vi "בדיקת זמן ניתוק הממסר 4.vi"(7 "resultUserPrompt":bool, 8 "error":errorcluster, 11 "Path for Log":path) -> (0 "error out":errorcluster, 1 "בטוח כן/לא":bool, 2 "בדיקת זמן ניתוק הממסר":dbl)   [LabVIEW 2015]
uses:
  <instrlib>/niDMM/nidmm.llb/niDMM Function.ctl
  <instrlib>/niDMM/nidmm.llb/niDMM Resolution in Digits.ctl
  <vilib>/DAQmx/write.llb/DAQmx Write (Digital Bool 1Line 1Point).vi
  <vilib>/DAQmx/create/channels.llb/DAQmx Create Channel (DO-Digital Output).vi
  <vilib>/DAQmx/miscellaneous.llb/DAQmx Fill In Error Info.vi
  <instrlib>/niDMM/nidmm.llb/niDMM Configure Measurement Digits.vi
panel:
  in  "התחל":bool
  # "Right-Click to\nexplain error"
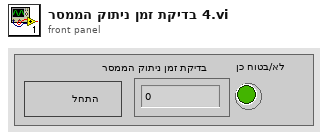
[diagram p1: front panel]
types:
  T1 = enum32{"Invalid", "Standard", "Closed", "Hidden", "Minimized", "Maximized"}
  T2 = typedef "niDMM Function.ctl" = enum16{"DC Volts", "AC Volts", "DC Current", "AC Current", "2-wire Resistance", "4-wire Resistance", "Diode", "Frequency", "Period", "AC Volts DC Coupled", "Capacitance", "Inductance", "Temperature"}
  T3 = typedef "niDMM Resolution in Digits.ctl" = dbl
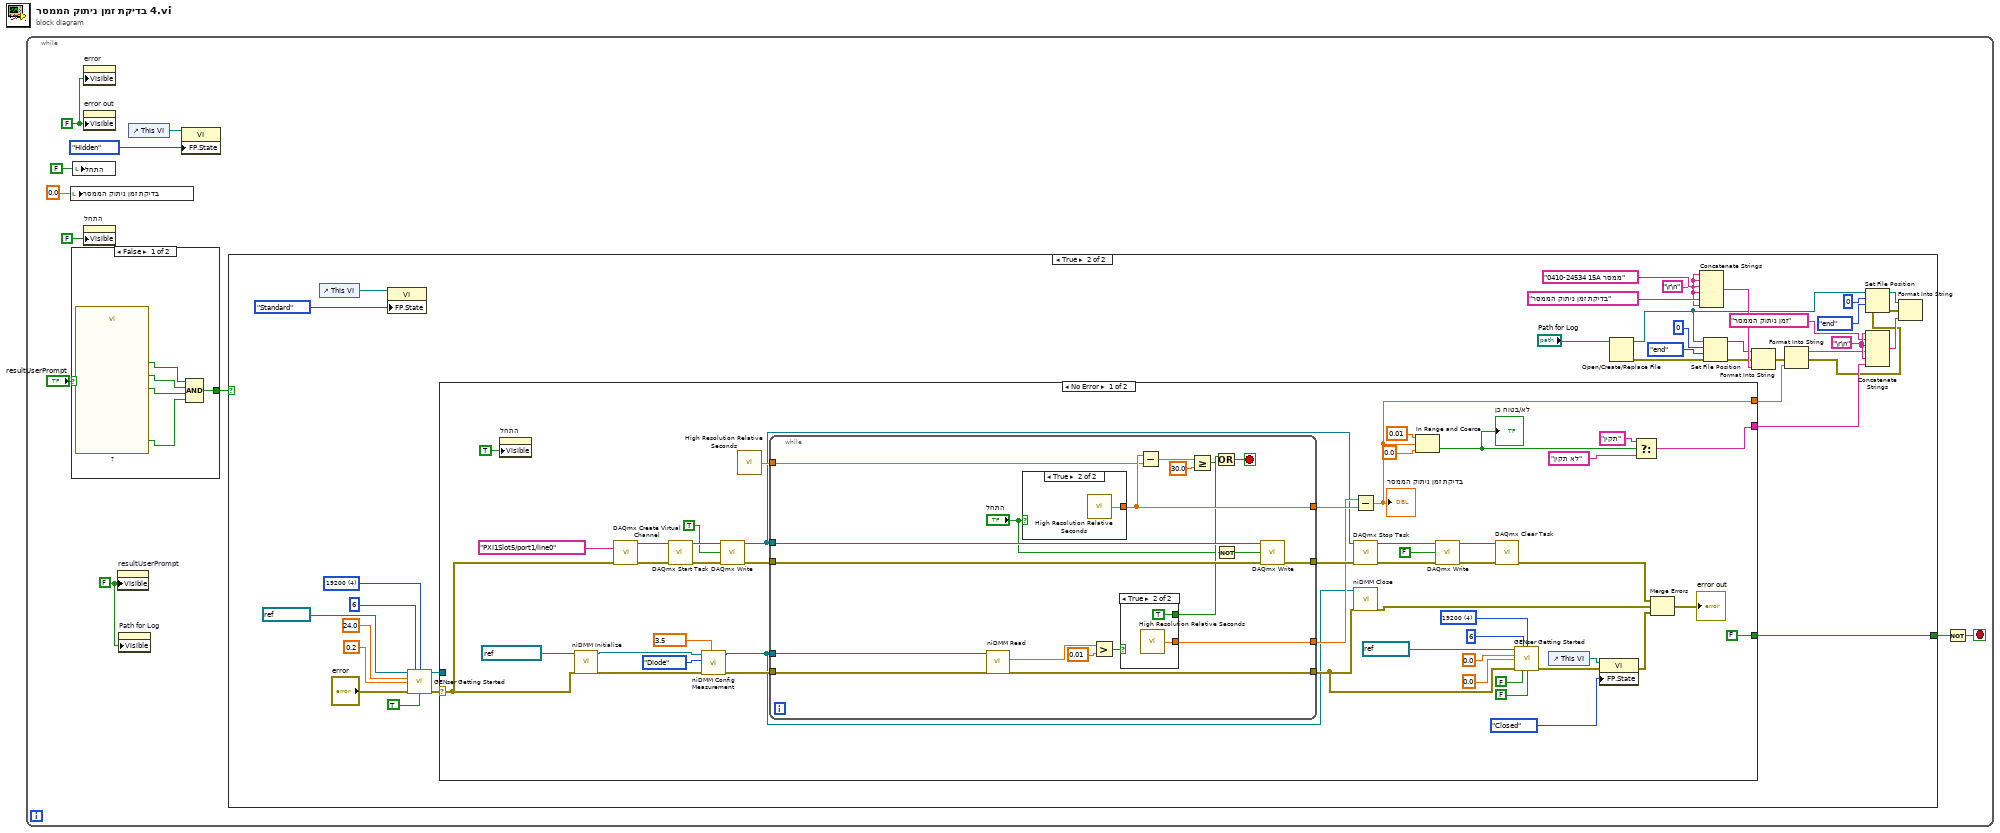
[diagram p0: block diagram]
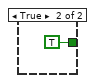
[diagram p2: hidden frame]
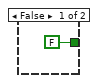
[diagram p3: hidden frame]
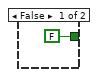
[diagram p4: hidden frame]
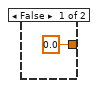
[diagram p5: hidden frame]
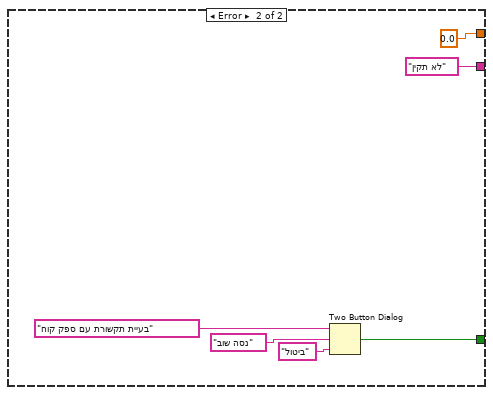
[diagram p6: hidden frame]
diagram:
  n1 = while {
    stop <- w10 stop-if-true
    w1 = FALSE ("Visible")
    w8 = FALSE ("Visible")
    n2 = local write "בדיקת זמן ניתוק הממסר"(0.0 ("זמן ניתוק הממסר")) -> ()
    n3 = case shown="False" "resultUserPrompt" {
      tunnel: [w16 TRUE] -> w11
      frame False {
        n4 = call "?"() -> ("הדקי הרב מודד"=w12:bool, "(מגע שלילי (מעטפת"=w13:bool, "A מגע חיובי"=w14:bool, "OK"=w15:bool)  [unwired: 15 in, 1 out]
        n5 = Compound Arithmetic op=AND(w15, w14, w13, w12) -> (w16:bool)
      }
      frame True {
      }
    }
    n6 = local write "התחל"(FALSE ("זמן ניתוק הממסר בטווח כן /לא")) -> ()
    n7 = property on="error" class="Clust (strict)"("Visible"=w8) -> ()  [unwired: 2 in, 2 out]
    n8 = property on="error out" class="Clust (strict)"("Visible"=w8) -> ()  [unwired: 2 in, 2 out]
    n9 = property on="התחל" class="Bool (strict)"("Visible"=FALSE) -> ()  [unwired: 2 in, 2 out]
    n10 = property on="resultUserPrompt" class="Bool (strict)"("Visible"=w1) -> ()  [unwired: 2 in, 2 out]
    n11 = property on="Path for Log" class="Path"("Visible"=w1) -> ()  [unwired: 2 in, 2 out]
    n12 = control-ref of="This VI"() -> (w7:refnum<vi>)
    n13 = property class="VI"(reference=w7, "FP.State"=T1."Hidden" ("Front Panel Window:State")) -> ()  [unwired: 1 in, 2 out]
    n14 = case shown="True" w11 {
      tunnel: [FALSE ("T button?") w46] -> w9
      frame False {
      }
      frame True {
        w27 = "\r\n"
        w35 = "\r\n"
        w50 = u16 4 items=["1200", "2400", "4800", "9600", "19200"] ("BAUD")
        n15 = control-ref of="This VI"() -> (w45:refnum<vi>)
        n16 = property class="VI"(reference=w45, "FP.State"=T1."Standard" ("Front Panel Window:State")) -> ()  [unwired: 1 in, 2 out]
        n17 = call "GENser Getting Started.vi"("VISA"=refnum<visa-resource-name> "COM6", "GEN Addr"=i16 6, "BAUD"=w50, "Voltage Limit"=24.0, "Current Limit"=0.2, "error"="error", "Output On (T)"=TRUE) -> ("VISA out"=w51:refnum<visa-resource-name>, "error out"=w42:errorcluster)  [unwired: 5 in, 2 out]
        n18 = case shown="No Error" w42 {
          selector: w42 -> [w56 _]
          tunnel: w51 -> [_ _]
          tunnel: [FALSE ("T button?") w129] -> w46
          tunnel: [w77 0.0] -> w21
          tunnel: [w73 "לא תקין"] -> w20
          frame No Error {
            w61 = T3 3.5 items=["3 1/2"=3.5, "4 1/2"=4.5, "5 1/2"=5.5, "6 1/2"=6.5, "7 1/2"=7.5] ("Resolution in Digits")
            w91 = u16 4 items=["1200", "2400", "4800", "9600", "19200"] ("BAUD")
            n19 = property on="התחל" class="Bool (strict)"("Visible"=TRUE) -> ()  [unwired: 2 in, 2 out]
            n20 = call <instrlib>:"niDMM Initialize.vi"("error in (no error)"=w56, "Instrument Descriptor"=refnum<k15> "PXI1Slot9") -> ("error out"=w58:errorcluster, "instrument handle out"=w59:refnum<k15>)  [unwired: 8 in]
            n21 = call-poly <vilib>:"DAQmx Create Virtual Channel.vi"("lines"=tag "PXI1Slot5/port1/line0", "error in"=w56) -> ("task out"=w70:refnum<k21>, "error out"=w71:errorcluster)  [unwired: 12 in]
            n22 = call <vilib>:"DAQmx Start Task.vi"("task/channels in"=w70, "error in"=w71) -> ("task out"=w67:refnum<k21>, "error out"=w66:errorcluster)  [unwired: 12 in]
            n23 = call-poly <instrlib>:"niDMM Config Measurement.vi"("Resolution in Digits"=w61, "error in (no error)"=w58, "Function"=niDMM_Function."Diode", "instrument handle"=w59) -> ("error out"=w60:errorcluster, "instrument handle out"=w55:refnum<k15>)  [unwired: 6 in]
            n24 = call-poly <vilib>:"DAQmx Write.vi"("task/channels in"=w67, "data"=TRUE, "error in"=w66) -> ("task out"=w54:refnum<k21>, "error out"=w65:errorcluster)  [unwired: 10 in, 1 out]
            n25 = call <vilib>:"High Resolution Relative Seconds.vi"() -> ("relative seconds"=w68:dbl)
            n26 = while {
              tunnel: [w116] -> w79
              tunnel: [w121] -> w78
              tunnel: [w120] -> w84
              tunnel: [w117] -> w57
              tunnel: w54 -> [w119]
              tunnel: w65 -> [w118]
              tunnel: w68 -> [w115]
              tunnel: w55 -> [w107]
              tunnel: w60 -> [w106]
              stop <- w112 stop-if-true
              n27 = call <instrlib>:"niDMM Read.vi"("error in (no error)"=w106, "instrument handle"=w107) -> ("error out"=w117:errorcluster, "Measurement"=w105:dbl)  [unwired: 7 in, 1 out]
              n28 = case shown="True" "התחל" {
                tunnel: [0.0 ("relative seconds") w126] -> w116
                frame False {
                }
                frame True {
                  n29 = call <vilib>:"High Resolution Relative Seconds.vi"() -> ("relative seconds"=w126:dbl)
                }
              }
              n30 = Greater?(x=w105, y=0.01) -> (0:w103:bool)
              n31 = case shown="True" w103 {
                tunnel: [_ w124] -> w121
                tunnel: [FALSE TRUE] -> w111
                frame False {
                }
                frame True {
                  n32 = call <vilib>:"High Resolution Relative Seconds.vi"() -> ("relative seconds"=w124:dbl)
                }
              }
              n33 = Subtract(x=w116, y=w115) -> (x-y=w114:dbl)
              n34 = Greater Or Equal?(x=w114, y=30.0) -> (x >= y?=w110:bool)
              n35 = Or(x=w111, y=w110) -> (x .or. y?=w112:bool)
              n36 = Not(x="התחל") -> (.not. x?=w109:bool)
              n37 = call-poly <vilib>:"DAQmx Write.vi"("task/channels in"=w119, "data"=w109, "error in"=w118) -> ("error out"=w120:errorcluster)  [unwired: 10 in, 2 out]
            }
            n38 = Subtract(x=w78, y=w79) -> (x-y=w77:dbl)
            "בדיקת זמן ניתוק הממסר" <- w77
            n39 = call <vilib>:"DAQmx Stop Task.vi"("task/channels in"=w54, "error in"=w84) -> ("task out"=w89:refnum<k21>, "error out"=w88:errorcluster)  [unwired: 12 in]
            n40 = call <instrlib>:"niDMM Close.vi"("error in (no error)"=w57, "instrument handle"=w55) -> ("error out"=w82:errorcluster)  [unwired: 9 in]
            n41 = In Range and Coerce(upper limit=0.01, x=w77, lower limit=0.0) -> (In Range?=w74:bool)  [unwired: 1 out]
            "בטוח כן/לא" <- w74
            n42 = call-poly <vilib>:"DAQmx Write.vi"("task/channels in"=w89, "data"=FALSE, "error in"=w88) -> ("task out"=w86:refnum<k21>, "error out"=w87:errorcluster)  [unwired: 10 in, 1 out]
            n43 = call <vilib>:"DAQmx Clear Task.vi"("task in"=w86, "error in"=w87) -> ("error out"=w83:errorcluster)  [unwired: 13 in]
            n44 = call "GENser Getting Started.vi"("VISA"=refnum<visa-resource-name> "COM6", "GEN Addr"=i16 6, "BAUD"=w91, "Voltage Limit"=0.0, "Current Limit"=0.0, "error"=w57, "Reset (T)"=FALSE ("Output On (T)"), "Output On (T)"=FALSE) -> ("error out"=w95:errorcluster)  [unwired: 4 in, 3 out]
            n45 = control-ref of="This VI"() -> (w97:refnum<vi>)
            n46 = property class="VI"(reference=w97, error in=w95, "FP.State"=T1."Closed" ("Front Panel Window:State")) -> (error out=w93:errorcluster)  [unwired: 1 out]
            n47 = Select(t="תקין", s=w74, f="לא תקין") -> (s? t:f=w73:string)
            n48 = Merge Errors(w83, w82, w93) -> (→"error out":errorcluster)
          }
          frame Error {
            n49 = Two Button Dialog(message="בעיית תקשורת עם ספק קוח", 1:"ביטול" ("F button name (\"Cancel\")"), 2:"נסה שוב" ("T button name (\"OK\")")) -> (T button?=w129:bool)
          }
        }
        n50 = Open/Create/Replace File(file path (use dialog)="Path for Log") -> (refnum out=w22:refnum<file>, error out=w23:errorcluster)  [unwired: 5 in, 1 out]
        n51 = Concatenate Strings(w35, w35, "0410-24534 15A ממסר", w35, "בדיקת זמן ניתוק הממסר", w35) -> (w39:string)
        n52 = Set File Position(offset (in bytes) (0)=i64 0, refnum=w22, from (0:start)=enum16{"start", "end", "current"}."end", error in=w23) -> (refnum out=w36:refnum<file>, error out=w34:errorcluster)
        n53 = Format Into String(initial string=w36, error in=w34, w39) -> (error out=w33:errorcluster)  [unwired: 1 in, 1 out]
        n54 = Format Into String(error in=w33, w21) -> (resulting string=w25:string, error out=w19:errorcluster)  [unwired: 2 in]
        n55 = Set File Position(offset (in bytes) (0)=i64 0, refnum=w22, from (0:start)=enum16{"start", "end", "current"}."end", error in=w19) -> (refnum out=w30:refnum<file>, error out=w31:errorcluster)
        n56 = Concatenate Strings(w27, "זמן ניתוק הממסר", w27, w25, w27, w20) -> (w32:string)
        n57 = Format Into String(initial string=w30, error in=w31, w32) -> ()  [unwired: 1 in, 2 out]
      }
    }
    n58 = Not(x=w9) -> (.not. x?=w10:bool)
  }
